vi "ArmTuningPathGenerator.vi"() -> (0 "Go":bool, 1 "Wrist Motion Profile":T1[](array[typedef]) {"Time (ms)" items=["TrajectoryDuration_0ms"=0, "TrajectoryDuration_5ms"=5, "TrajectoryDuration_10ms"=10, "TrajectoryDuration_20ms"=20, "TrajectoryDuration_30ms"=30, "TrajectoryDuration_40ms"=40, "TrajectoryDuration_50ms"=50, "TrajectoryDuration_100ms"=100]}, 2 "Extension Motion Profile":T1[](array[typedef]) {"Time (ms)" items=["TrajectoryDuration_0ms"=0, "TrajectoryDuration_5ms"=5, "TrajectoryDuration_10ms"=10, "TrajectoryDuration_20ms"=20, "TrajectoryDuration_30ms"=30, "TrajectoryDuration_40ms"=40, "TrajectoryDuration_50ms"=50, "TrajectoryDuration_100ms"=100]}, 3 "Shoulder Motion Profile":T1[](array[typedef]) {"Time (ms)" items=["TrajectoryDuration_0ms"=0, "TrajectoryDuration_5ms"=5, "TrajectoryDuration_10ms"=10, "TrajectoryDuration_20ms"=20, "TrajectoryDuration_30ms"=30, "TrajectoryDuration_40ms"=40, "TrajectoryDuration_50ms"=50, "TrajectoryDuration_100ms"=100]})   [LabVIEW 2018]
uses:
  ArgosLib/Signal Processing/TypeDefs/EdgeDetector_Type.ctl
  ArgosLib/ArgosLib.lvlib
  <vilib>/Rock Robotics/WPI/ThirdParty/Phoenix-LabVIEW/Motor Controller/Controls/CTRE_Phoenix_MotorControl_TrajectoryPointTimeDur.ctl
  ArgosLib/MotionProfiling/TypeDefs/TrajectoryPoint.ctl
  ArgosLib/MotionProfiling/TypeDefs/MotionProfileGeneratorParams.ctl
panel:
  in  "Preview Only":bool
  out "Wrist Motion Profile Graph":T3(graph)
  in  "Enable Wrist":bool
  in  "Start Wrist Angle":dbl
  in  "End Wrist Angle":dbl
  in  "Enable extension":bool
  in  "Enable Shoulder":bool
  out "Extension Motion Profile Graph":T3(graph)
  out "Shoulder Motion Profile Graph":T3(graph)
  in  "MotionProfileGeneratorParameters":T4={"Trajectory Point Interval (ms)"=10, "Maximum Travel Speed (units/s)"=500.0, "Velocity Ramp Time (ms)"=400.0, "Acceleration Ramp Time (ms)"=200.0} {"Acceleration Ramp Time (ms)" min=1.0; "Velocity Ramp Time (ms)" min=1.0; "Maximum Travel Speed (units/s)" min=0.0; "Trajectory Point Interval (ms)" items=["TrajectoryDuration_0ms"=0, "TrajectoryDuration_5ms"=5, "TrajectoryDuration_10ms"=10, "TrajectoryDuration_20ms"=20, "TrajectoryDuration_30ms"=30, "TrajectoryDuration_40ms"=40, "TrajectoryDuration_50ms"=50, "TrajectoryDuration_100ms"=100]}
  in  "Reverse Direction":bool
  in  "Send Motion Profiles":bool
  in  "End Extension":dbl
  in  "Start Extension":dbl
  in  "End Shoulder Angle":dbl
  in  "Start Shoulder Angle":dbl
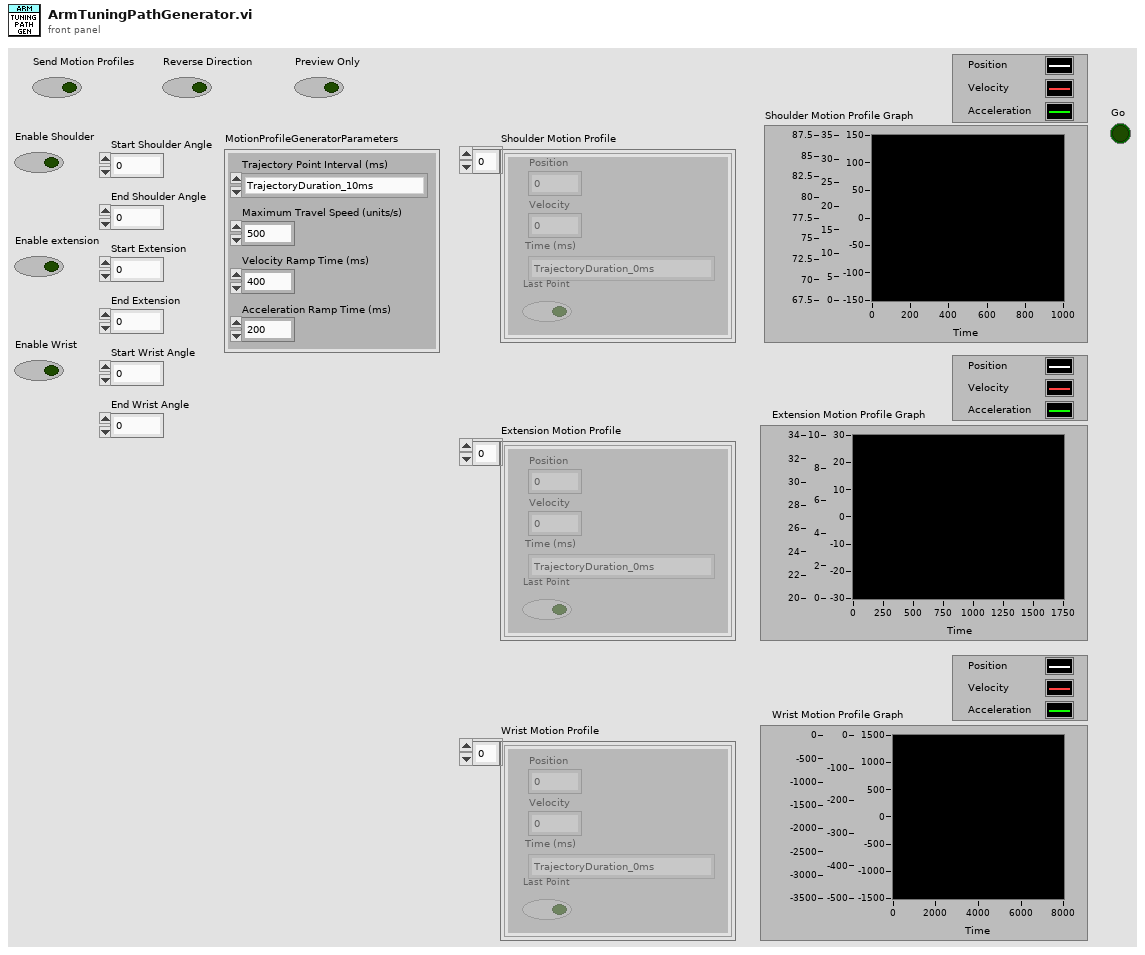
[diagram p1: front panel]
types:
  T1 = typedef "TrajectoryPoint.ctl" = cluster{"Position ":dbl, "Velocity ":dbl, "Time (ms)":T2, "Last Point":bool}
  T2 = typedef "CTRE_Phoenix_MotorControl_TrajectoryPointTimeDur.ctl" = i32
  T3 = cluster{dbl, "Trajectory Point Interval (ms)":i32, dbl[][]}
  T4 = typedef "MotionProfileGeneratorParams.ctl" = cluster{"Trajectory Point Interval (ms)":T2, "Maximum Travel Speed (units/s)":dbl, "Velocity Ramp Time (ms)":dbl, "Acceleration Ramp Time (ms)":dbl}
  T5 = typedef "ArgosLib.lvlib/EdgeDetector_Type.ctl" = enum16{"RisingEdge", "FallingEdge", "Both"}
  T6 = cluster{dbl, "Trajectory Point Interval (ms)":T2, dbl[][]}
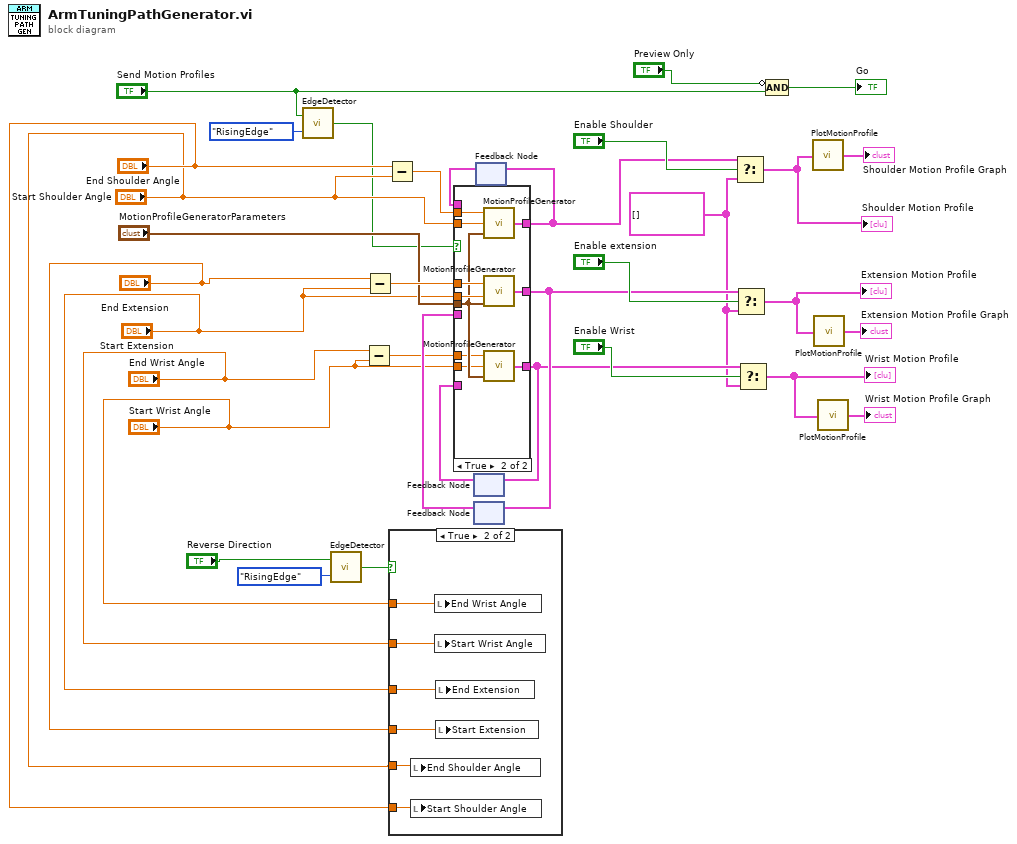
[diagram p0: block diagram]
diagram:
  w6 = T1[] [] ("f")
  n1 = call "EdgeDetector.vi"("DetectorType"=EdgeDetector_Type."RisingEdge", "Input"="Send Motion Profiles") -> ("Edge"=w14:bool)
  n2 = call "EdgeDetector.vi"("DetectorType"=EdgeDetector_Type."RisingEdge", "Input"="Reverse Direction") -> ("Edge"=w26:bool)
  n3 = Subtract(x="End Wrist Angle", y="Start Wrist Angle") -> (x-y=w9:dbl)
  n4 = Subtract(x="End Extension", y="Start Extension") -> (x-y=w33:dbl)
  n5 = Subtract(x="End Shoulder Angle", y="Start Shoulder Angle") -> (x-y=w34:dbl)
  n6 = case shown="True" w26 {
    tunnel: "End Shoulder Angle" -> [_ w40]
    tunnel: "Start Shoulder Angle" -> [_ w39]
    tunnel: "End Extension" -> [_ w38]
    tunnel: "Start Extension" -> [_ w37]
    tunnel: "End Wrist Angle" -> [_ w36]
    tunnel: "Start Wrist Angle" -> [_ w35]
    frame False {
    }
    frame True {
      n7 = local write "End Shoulder Angle"(w39) -> ()
      n8 = local write "Start Shoulder Angle"(w40) -> ()
      n9 = local write "End Wrist Angle"(w35) -> ()
      n10 = local write "Start Wrist Angle"(w36) -> ()
      n11 = local write "End Extension"(w37) -> ()
      n12 = local write "Start Extension"(w38) -> ()
    }
  }
  n13 = feedback #1() -> (w12:T1[])  [unwired: 1 in]
  n14 = feedback #2() -> (w17:T1[])  [unwired: 1 in]
  n15 = feedback #3() -> (w15:T1[])  [unwired: 1 in]
  n16 = case shown="True" w14 {
    tunnel: w34 -> [_ w53]
    tunnel: w33 -> [_ w52]
    tunnel: "MotionProfileGeneratorParameters" -> [_ w47]
    tunnel: "Start Extension" -> [_ w51]
    tunnel: "Start Shoulder Angle" -> [_ w50]
    tunnel: [w42 w49] -> w16
    tunnel: [w43 w48] -> w18
    tunnel: w17 -> [w43 _]
    tunnel: w15 -> [w42 _]
    tunnel: [w41 w46] -> w7
    tunnel: w12 -> [w41 _]
    tunnel: w9 -> [_ w45]
    tunnel: "Start Wrist Angle" -> [_ w44]
    frame False {
    }
    frame True {
      n17 = call "MotionProfileGenerator.vi"("MotionProfileGeneratorParameters"=w47, "Starting Position (units)"=w50, "Travel Distance (units)"=w53) -> ("Trajectory Points"=w49:T1[])
      n18 = call "MotionProfileGenerator.vi"("MotionProfileGeneratorParameters"=w47, "Starting Position (units)"=w51, "Travel Distance (units)"=w52) -> ("Trajectory Points"=w48:T1[])
      n19 = call "MotionProfileGenerator.vi"("MotionProfileGeneratorParameters"=w47, "Starting Position (units)"=w44, "Travel Distance (units)"=w45) -> ("Trajectory Points"=w46:T1[])
    }
  }
  n20 = feedback-in #1(w7) -> ()
  n21 = feedback-in #2(w18) -> ()
  n22 = feedback-in #3(w16) -> ()
  n23 = Select(t=w16, s="Enable Shoulder", f=w6) -> (s? t:f=w19:T1[])
  "Shoulder Motion Profile" <- w19
  n24 = Select(t=w18, s="Enable extension", f=w6) -> (s? t:f=w20:T1[])
  "Extension Motion Profile" <- w20
  n25 = Select(t=w7, s="Enable Wrist", f=w6) -> (s? t:f=w4:T1[])
  "Wrist Motion Profile" <- w4
  n26 = Compound Arithmetic op=AND(invert "Preview Only", "Send Motion Profiles") -> (→"Go":bool)
  n27 = call "PlotMotionProfile.vi"("Trajectory Points"=w19) -> ("MotionProfileGraph"=→"Shoulder Motion Profile Graph":T6)
  n28 = call "PlotMotionProfile.vi"("Trajectory Points"=w20) -> ("MotionProfileGraph"=→"Extension Motion Profile Graph":T6)
  n29 = call "PlotMotionProfile.vi"("Trajectory Points"=w4) -> ("MotionProfileGraph"=→"Wrist Motion Profile Graph":T6)
